vi "Actor Core.vi"(8 "error in":errorcluster, 11 "Splitter Settings UI in":refnum<class "Splitter Settings UI.lvclass">) -> (0 "error out":errorcluster, 3 "Actor out":refnum<class "Actor.lvclass">)   [LabVIEW 2017, in "Splitter Settings UI.lvlib" / "Splitter Settings UI.lvclass"]
doc: "The user interface for this panel.\n\n----\nPlease see the following web address for additional documentation and tutorial information:\nhttp://www.mooregoodideas.com/mgi-panel-manager/\n\nAuthor: Derek Trepanier\n\nCopyright (c) 2018, Moore Good Ideas, Inc.\n\nAll rights reserved.\n\nRedistribution and use in source and binary forms, with or without modification, are permitted provided that the following conditions are met:\n\n * Redistributions of source code must retain the above copyright notice, this list of conditions and the following disclaimer.\n * Redistributions in binary form must reproduce the above copyright notice, this list of conditions and the following disclaimer in the documentation and/or other materials provided with the distribution.\n * Neither the name of Moore Good Ideas, Inc. nor the names of its contributors may be used to endorse or promote products derived from this software without specific prior written permission.\n\nTHIS SOFTWARE IS PROVIDED BY THE COPYRIGHT HOLDERS AND CONTRIBUTORS \"AS IS\" AND ANY EXPRESS OR IMPLIED WARRANTIES, INCLUDING, BUT NOT LIMITED TO, THE IMPLIED WARRANTIES OF MERCHANTABILITY AND FITNESS FOR A PARTICULAR PURPOSE ARE DISCLAIMED. IN NO EVENT SHALL THE COPYRIGHT OWNER OR CONTRIBUTORS BE LIABLE FOR ANY DIRECT, INDIRECT, INCIDENTAL, SPECIAL, EXEMPLARY, OR CONSEQUENTIAL DAMAGES (INCLUDING, BUT NOT LIMITED TO, PROCUREMENT OF SUBSTITUTE GOODS OR SERVICES; LOSS OF USE, DATA, OR PROFITS; OR BUSINESS INTERRUPTION) HOWEVER CAUSED AND ON ANY THEORY OF LIABILITY, WHETHER IN CONTRACT, STRICT LIABILITY, OR TORT (INCLUDING NEGLIGENCE OR OTHERWISE) ARISING IN ANY WAY OUT OF THE USE OF THIS SOFTWARE, EVEN IF ADVISED OF THE POSSIBILITY OF SUCH DAMAGE."
uses:
  Splitter Settings UI.lvclass
  C:/Program Files (x86)/National Instruments/LabVIEW 2017/vi.lib/MNProjects/Panel Manager/panel-actors/Source/Panel Actor/Panel Actor.lvclass
  C:/Program Files (x86)/National Instruments/LabVIEW 2017/vi.lib/ActorFramework/Actor/Actor.lvclass
  <vilib>/ActorFramework/Actor/Actor.lvclass
  Splitter/Splitter.lvclass
  <vilib>/ActorFramework/Actor/Actor.lvclass/Actor.ctl
  <vilib>/ActorFramework/Message Enqueuer/Message Enqueuer.lvclass/Message Enqueuer.ctl
  Splitter Settings UI.lvclass/Splitter Settings UI.ctl
  Splitter Settings UI Messages/Set Cursor Busy State Msg/Set Cursor Busy State Msg.lvclass/Set Cursor Busy State Msg.ctl
  <vilib>/ActorFramework/Message Enqueuer/Init from Existing Queue.vi
  <vilib>/ActorFramework/Message Enqueuer/Enqueue.vi
  Pane Relief Main UI/Pane Relief Main UI Messages/Panel Object Settings Changed Msg/Panel Object Settings Changed Msg.lvclass
  C:/Program Files (x86)/National Instruments/LabVIEW 2017/vi.lib/ActorFramework/Message/Message.lvclass
  Splitter Settings UI Messages/Set Cursor Busy State Msg/Set Cursor Busy State Msg.lvclass
  <vilib>/ActorFramework/Message Priority Queue/Priority Enqueue.vi
  <vilib>/ActorFramework/Message Enqueuer/Message Enqueuer.lvclass
  <vilib>/MNProjects/Panel Manager/panel-actors/Source/Panel Actor/Panel Actor.lvclass
panel:
  in  "Label":string
  in  "Size":i32 min=0
  in  "Color":u32(colorbox)
  in  "Locked":bool
  in  "Sizing":u16(ring) items=["Sticks Top", "Sticks Bottom", "Proportional"]
  in  "Position":i32
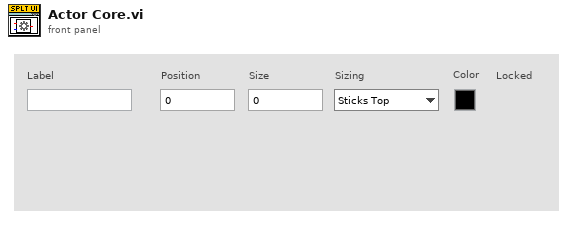
[diagram p1: front panel]
types:
  T1 = cluster{"Event Registration Refnum":refnum<event-registration>, "Pnl Actor":refnum<event-registration>}
  T2 = typedef "Splitter Sizing--Enum.ctl" = enum16{"Sticks Top/Left", "Sticks Bottom/Right", "Proportional"}
  T3 = typedef "Splitter Orientation--Enum.ctl" = enum16{"Vertical", "Horizontal"}
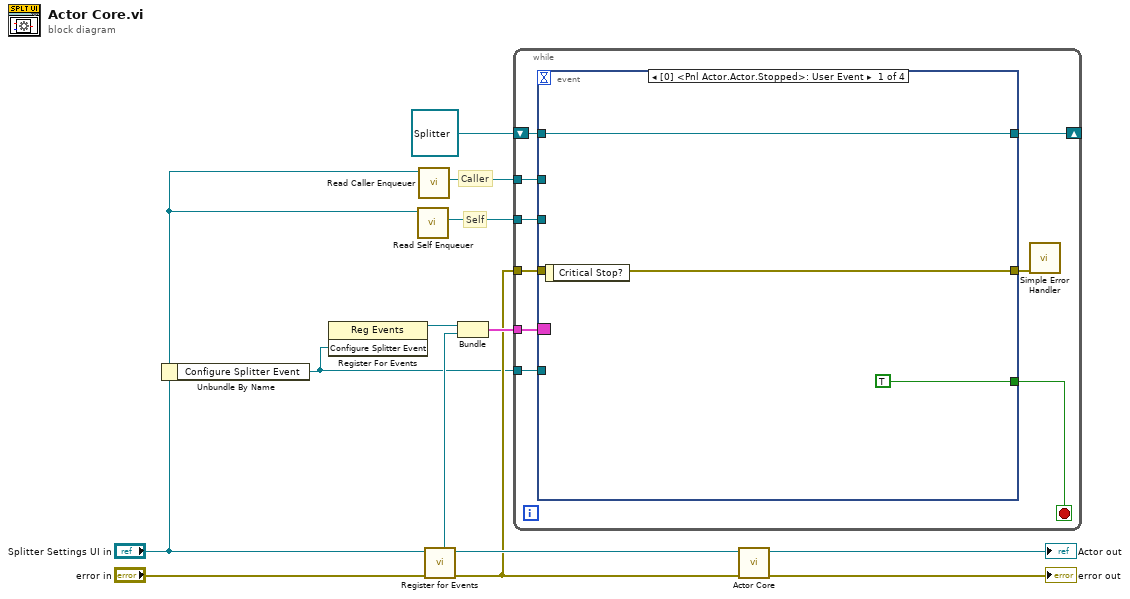
[diagram p0: block diagram]
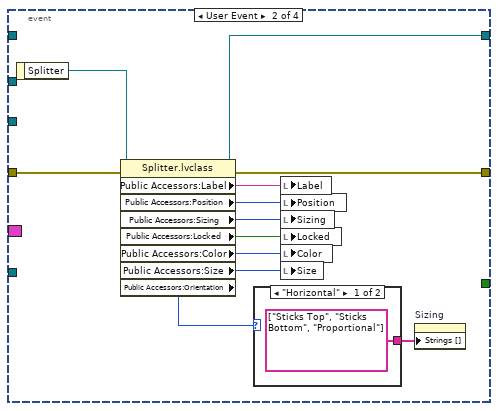
[diagram p2: hidden frame]
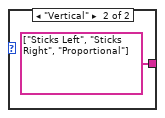
[diagram p3: hidden frame]
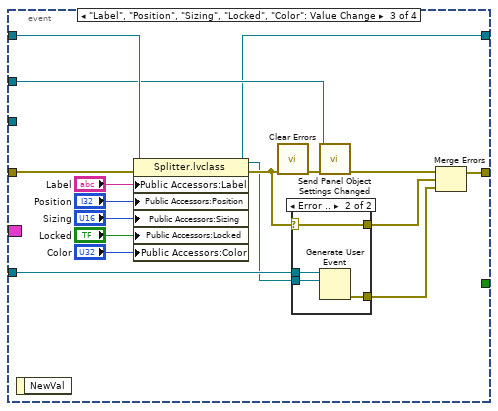
[diagram p4: hidden frame]
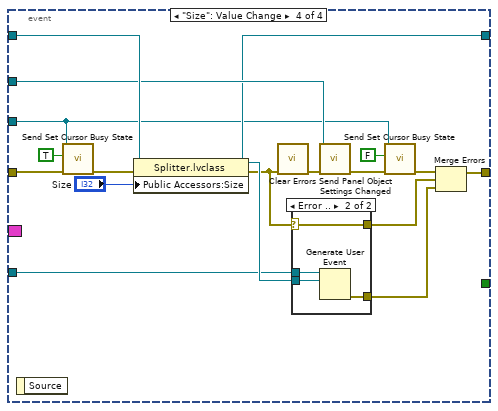
[diagram p6: hidden frame]
diagram:
  # "Self"
  # "Caller"
  n1 = Unbundle By Name("Splitter Settings UI in") -> ("Configure Splitter Event"=w3:refnum<user-event>)
  n2 = register-events(w3) -> (reference out=w9:refnum<event-registration>)  [unwired: 2 in, 1 out]
  n3 = call <vilib>:"Read Self Enqueuer.vi"("Actor"="Splitter Settings UI in") -> ("Self Enqueuer"=w2:refnum<class "Message Enqueuer.lvclass">)  [unwired: 10 in]
  n4 = call <vilib>:"Read Caller Enqueuer.vi"("Actor"="Splitter Settings UI in") -> ("Caller Enqueuer"=w4:refnum<class "Message Enqueuer.lvclass">)  [unwired: 10 in]
  n5 = call <vilib>:"Register for Events.vi"("Error In"="error in", "Panel Actor in"="Splitter Settings UI in") -> ("Error Out"=w5:errorcluster, "Panel Actor out"=w11:refnum<class "Splitter Settings UI.lvclass">, "Pnl Actor"=w8:refnum<event-registration>)  [unwired: 5 in, 2 out]
  n6 = Bundle("Event Registration Refnum"=w9, "Pnl Actor"=w8) -> (w7:T1)  [unwired: 1 in]
  n7 = while {
    tunnel: w7 -> [w22]
    shift-right: [w20] -> _
    shift-left: refnum<class "Splitter.lvclass"> refnum ("Splitter.lvclass") -> [w19]
    tunnel: w4 -> [w17]
    tunnel: w5 -> [w18]
    tunnel: w3 -> [w15]
    tunnel: w2 -> [w14]
    stop <- w21 stop-if-true
    n8 = event shown="[0] <Pnl Actor.Actor.Stopped>: User Event" {
      selector: w22 -> [_ _ _ _]
      dyn-events: _ -> [_ _ _ _]
      timeout: _ -> [_ _ _ _]
      tunnel: [TRUE _ _ _] -> w21
      tunnel: [w25 w30 w41 w70] -> w20
      tunnel: w19 -> [w25 _ w49 w77]
      tunnel: w18 -> [w24 w32 w50 w65]
      tunnel: [w24 w31 w45 w74] -> w16
      tunnel: w17 -> [_ _ w47 w73]
      tunnel: w15 -> [_ _ w42 w68]
      tunnel: w14 -> [_ _ _ w63]
      event User Event {
        n9 = event-data() -> ()  [unwired: 1 in, 1 out]
      }
      event User Event {
        n10 = event-data() -> ("Splitter"=w29:refnum<class "Splitter.lvclass">)  [unwired: 1 in]
        n11 = property class="Splitter.lvclass"(reference=w29, error in=w32) -> (reference out=w30:refnum<class "Splitter.lvclass">, error out=w31:errorcluster, "Public Accessors:Label"=w37:string, "Public Accessors:Position"=w36:i32, "Public Accessors:Sizing"=w35:T2, "Public Accessors:Locked"=w34:bool, "Public Accessors:Color"=w33:u32, "Public Accessors:Size"=w28:i32, "Public Accessors:Orientation"=w27:T3)
        n12 = case shown="\"Horizontal\"" w27 {
          tunnel: [string[] ["Sticks Top", "Sticks Bottom", "Proportional"] ("Strings []") string[] ["Sticks Left", "Sticks Right", "Proportional"] ("Strings []")] -> w26
          frame "Horizontal" {
          }
          frame "Vertical" {
          }
        }
        n13 = local write "Label"(w37) -> ()
        n14 = local write "Position"(w36) -> ()
        n15 = local write "Sizing"(w35) -> ()
        n16 = local write "Locked"(w34) -> ()
        n17 = local write "Color"(w33) -> ()
        n18 = local write "Size"(w28) -> ()
        n19 = property on="Sizing" class="Ring (strict)"("Strings []"=w26) -> ()  [unwired: 2 in, 2 out]
      }
      event "Label", "Position", "Sizing", "Locked", "Color": Value Change {
        n20 = event-data() -> ()  [unwired: 1 in, 1 out]
        n21 = property class="Splitter.lvclass"(reference=w49, error in=w50, "Public Accessors:Label"="Label", "Public Accessors:Position"="Position", "Public Accessors:Sizing"="Sizing", "Public Accessors:Locked"="Locked", "Public Accessors:Color"="Color") -> (reference out=w41:refnum<class "Splitter.lvclass">, error out=w43:errorcluster)
        n22 = call <vilib>:"Clear Errors.vi"("error in (no error)"=w43) -> ("error out"=w48:errorcluster)  [unwired: 5 in, 1 out]
        n23 = case shown="Error .." w43 {
          selector: w43 -> [w56 w60]
          tunnel: [w56 w60] -> w44
          tunnel: w42 -> [_ w59]
          tunnel: w41 -> [_ w58]
          tunnel: [_ w57] -> w40
          frame No Error {
          }
          frame Error {
            n24 = Generate User Event(user event=w59, event data cluster=w58) -> (error out=w57:errorcluster)  [unwired: 2 in, 1 out]
          }
        }
        n25 = call "Send Panel Object Settings Changed.vi"("error in (no error)"=w48, "Message Enqueuer"=w47) -> ("error out"=w46:errorcluster)  [unwired: 8 in, 1 out]
        n26 = Merge Errors(w46, w44, w40) -> (w45:errorcluster)
      }
      event "Size": Value Change {
        n27 = event-data() -> ()  [unwired: 1 in, 1 out]
        n28 = call "Send Set Cursor Busy State.vi"("error in (no error)"=w65, "Busy?"=TRUE, "Message Enqueuer"=w63) -> ("error out"=w66:errorcluster)  [unwired: 7 in, 1 out]
        n29 = property class="Splitter.lvclass"(reference=w77, error in=w66, "Public Accessors:Size"="Size") -> (reference out=w70:refnum<class "Splitter.lvclass">, error out=w69:errorcluster)
        n30 = call <vilib>:"Clear Errors.vi"("error in (no error)"=w69) -> ("error out"=w75:errorcluster)  [unwired: 5 in, 1 out]
        n31 = case shown="Error .." w69 {
          selector: w69 -> [w78 w82]
          tunnel: [w78 w82] -> w72
          tunnel: w68 -> [_ w81]
          tunnel: w70 -> [_ w80]
          tunnel: [_ w79] -> w71
          frame No Error {
          }
          frame Error {
            n32 = Generate User Event(user event=w81, event data cluster=w80) -> (error out=w79:errorcluster)  [unwired: 2 in, 1 out]
          }
        }
        n33 = call "Send Panel Object Settings Changed.vi"("error in (no error)"=w75, "Message Enqueuer"=w73) -> ("error out"=w62:errorcluster)  [unwired: 8 in, 1 out]
        n34 = call "Send Set Cursor Busy State.vi"("error in (no error)"=w62, "Busy?"=FALSE, "Message Enqueuer"=w63) -> ("error out"=w61:errorcluster)  [unwired: 7 in, 1 out]
        n35 = Merge Errors(w61, w72, w71) -> (w74:errorcluster)
      }
    }
    n36 = call <vilib>:"Simple Error Handler.vi"("error in (no error)"=w16) -> ()  [unwired: 4 in, 5 out]
  }
  n37 = call-parent "Actor Core.vi"("error in"=w5, "Panel Actor in"=w11) -> ("error out"=→"error out":errorcluster, "Actor out"=→"Actor out":refnum<class "Actor.lvclass">)  [unwired: 8 in]
